vi "_Get Simulation Spectrum.vi"(4 "ErrorIn":errorcluster, 5 "Index Array":i64[][](array[numeric]), 6 "RetTime(mS)":i32=1, 7 "FileRefIn":refnum<file>) -> (0 "ErrorOut":errorcluster, 1 "TIC":u32, 2 "Spectrum":i32[](array[numeric]), 3 "FileRefOut":refnum<file>)   [LabVIEW 2015]
panel:
  out "RemainderTime":i64
  out "Offset":i64
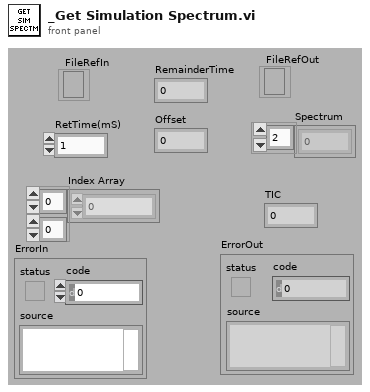
[diagram p1: front panel]
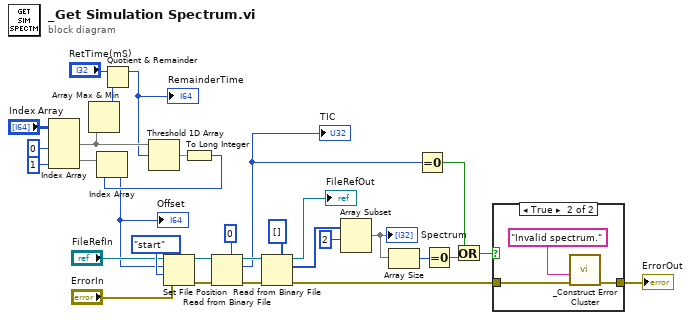
[diagram p0: block diagram]
diagram:
  n1 = Index Array(array="Index Array", index (col) #1=0 ("disabled index (col)"), index (col) #2=1 ("index (col)")) -> (element #1=w28:i64[], element #2=w13:i64[])  [unwired: 2 in]
  n2 = Array Max & Min(array=w28) -> (max value=w26:i64)  [unwired: 3 out]
  n3 = Quotient & Remainder(x="RetTime(mS)", y=w26) -> (x-y*floor(x/y)=w1:i64)  [unwired: 1 out]
  "RemainderTime" <- w1
  n4 = Threshold 1D Array(2:w1, 3:w28) -> (0:w29:dbl)  [unwired: 1 in]
  n5 = To Long Integer(number=w29) -> (32bit integer=w12:i32)
  n6 = Index Array(array=w13, index=w12) -> (element=w11:i64)
  "Offset" <- w11
  n7 = Set File Position(offset (in bytes) (0)=w11, refnum="FileRefIn", from (0:start)=enum16{"start", "end", "current"}."start" ("pos mode (0:2)"), error in="ErrorIn") -> (refnum out=w21:refnum<file>, error out=w20:errorcluster)
  n8 = Read from Binary File(5:u32 0, 8:w20, 11:w21) -> (0:w23:errorcluster, 2:w7:u32, 3:w24:refnum<file>)  [unwired: 4 out]
  "TIC" <- w7
  n9 = Read from Binary File(5:u32[] [] ("Spectrum"), 8:w23, 11:w24) -> (0:w3:errorcluster, 2:w15:u32[], 3:→"FileRefOut":refnum<file>)  [unwired: 4 out]
  n10 = Array Subset(array=w15, index=2) -> (w9:u32[])  [unwired: 1 in]
  "Spectrum" <- w9
  n11 = Array Size(array=w9) -> (size(s)=w8:i32)
  n12 = Equal To 0?(x=w7) -> (x = 0?=w5:bool)
  n13 = Equal To 0?(x=w8) -> (x = 0?=w6:bool)
  n14 = Or(x=w5, y=w6) -> (x .or. y?=w4:bool)
  n15 = case shown="True" w4 {
    tunnel: w3 -> [w32 w34]
    tunnel: [w32 w33] -> w2
    frame False {
    }
    frame True {
      n16 = call "_Construct Error Cluster.vi"("error in"=w34, "reason"="Invalid spectrum.") -> ("error out"=w33:errorcluster)  [unwired: 2 in, 3 out]
    }
  }
  "ErrorOut" <- w2
